vi "Set VI Reentrancy.vi"(6 "Reentrancy Type":T1(ring), 8 "error in (no error)":errorcluster, 9 "Is Reentrant":bool, 10 "VI Name":string, 11 "Application Reference":refnum<vi>) -> (0 "error out":errorcluster)   [LabVIEW 2013, in "LVTM.lvlib"]
uses:
  LVTM.lvlib
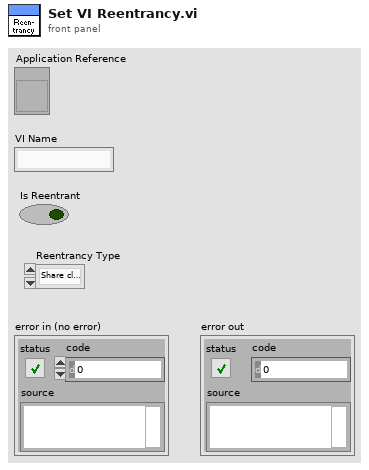
[diagram p1: front panel]
types:
  T1 = enum16{"Share clones between instances", "Preallocate clone for each instance"}
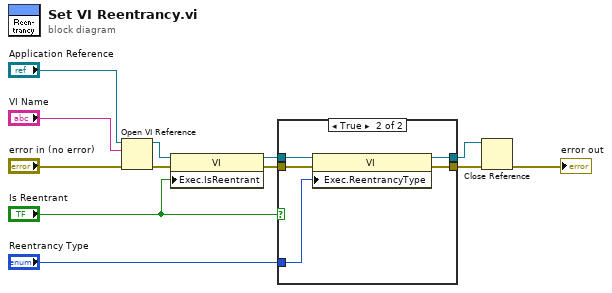
[diagram p0: block diagram]
diagram:
  n1 = Open VI Reference(application reference (local)="Application Reference", vi path="VI Name", error in (no error)="error in (no error)") -> (vi reference=w11:refnum<vi>, error out=w10:errorcluster)  [unwired: 3 out]
  n2 = property class="VI"(reference=w11, error in=w10, "Exec.IsReentrant"="Is Reentrant") -> (reference out=w6:refnum<vi>, error out=w4:errorcluster)
  n3 = case shown="True" "Is Reentrant" {
    tunnel: w6 -> [w14 w19]
    tunnel: [w14 w18] -> w5
    tunnel: [w13 w17] -> w1
    tunnel: w4 -> [w13 w16]
    tunnel: "Reentrancy Type" -> [_ w15]
    frame False {
    }
    frame True {
      n4 = property class="VI"(reference=w19, error in=w16, "Exec.ReentrancyType"=w15) -> (reference out=w18:refnum<vi>, error out=w17:errorcluster)
    }
  }
  n5 = Close Reference(reference=w5, error in (no error)=w1) -> (error out=→"error out":errorcluster)
